vi "SIM Rosenbrock manager.vi"(1 "Simulation data":T1={"continuous integrator"=enum."RK 1 (Euler)", "initial time"=0.0, "final time"=6.0, "step size"=0.0, "proposed step size"=0.001, "max step size"=1e-06, "min step size"=0.0, "discrete time step"=0.0, "max step ratio"=3.0, "Diag Eval Stage"=enum."Major Substep", "Substep Index"=0, "Timestep Index"=10.0, "simulation time"=0.0, "current timestep base"=0.1, "proposed step time"=0.0, "absolute tolerance"=0.0, "relative tolerance"=0.0, "step accepted?"=FALSE, "step complete?"=FALSE, "Halt?"=FALSE, "reset integrator?"=FALSE, "machine epsilon"=1.0, "min float"=0.0, "error"={"status"=FALSE, "code"=0, "source"=""}, "Method Order"=0, "Finished Late [i-1]"=FALSE, "Discrete step?"=FALSE, "NaN and Inf check?"=FALSE, "Final Timestep Index"=0.0, "(maj+disc)or(init)?"=FALSE, "Full Solver Reset"=TRUE, "Execution Mode"=enum."Simulate to Completion", "check vector sizes?"=FALSE, "solver handles zc?"=FALSE, "Simulation Registry"={"Current Idx"=0, "Node Tags"=[], "Node Headers"=[], "Node Data"=[], "Cont State data"={"inputs"=[], "outputs"=[], "reset"=[], "lower limits"=[], "upper limits"=[], "limit types"=[], "reset types"=[], "initial conditions"=[], "reset I.C."=[], "limited?"=[], "State Names"=[]}, "DiscreteInfo"={"tick period (sec)"=0.0, "time (ticks)"=0, "fire?"=[], "registry"={"period (sec)"=[], "skew (sec)"=[], "period (tick)"=[], "skew (tick)"=[]}, "discrete \nblocks?"=FALSE, "steps per tick"=0.0, "steps to tick"=0.0, "discrete \ntick?"=FALSE}, "Disc State data"={"Disc States"=[], "State Names"=[]}, "Registry Error"={"Error Block ID"=0, "code"=0}, "ZC Indices"=[]}, "variable step solver?"=FALSE, "First Substep?"=FALSE, "Continuous States?"=FALSE} {"min float" format="%.1e"; "proposed step size" format="%.1e"; "proposed step time" format="%.1e"; "max step ratio" format="%.1e"; "min step size" format="%.1e"; "machine epsilon" format="%.1e"; "discrete time step" format="%.1e"; "max step size" format="%.1e"; "current timestep base" format="%.1e"; "final time" format="%.1e"; "simulation time" format="%.1e"; "relative tolerance" format="%.1e"; "absolute tolerance" format="%.1e"; "Substep Index" format="%.1e"; "step size" format="%.1e"; "initial time" format="%.1e"}) -> (0 "Simulation data out":T1={"continuous integrator"=enum."RK 1 (Euler)", "initial time"=0.0, "final time"=6.0, "step size"=0.0, "proposed step size"=0.001, "max step size"=1e-06, "min step size"=0.0, "discrete time step"=0.0, "max step ratio"=3.0, "Diag Eval Stage"=enum."Major Substep", "Substep Index"=0, "Timestep Index"=10.0, "simulation time"=0.0, "current timestep base"=0.1, "proposed step time"=0.0, "absolute tolerance"=0.0, "relative tolerance"=0.0, "step accepted?"=FALSE, "step complete?"=FALSE, "Halt?"=FALSE, "reset integrator?"=FALSE, "machine epsilon"=1.0, "min float"=0.0, "error"={"status"=FALSE, "code"=0, "source"=""}, "Method Order"=0, "Finished Late [i-1]"=FALSE, "Discrete step?"=FALSE, "NaN and Inf check?"=FALSE, "Final Timestep Index"=0.0, "(maj+disc)or(init)?"=FALSE, "Full Solver Reset"=TRUE, "Execution Mode"=enum."Simulate to Completion", "check vector sizes?"=FALSE, "solver handles zc?"=FALSE, "Simulation Registry"={"Current Idx"=0, "Node Tags"=[], "Node Headers"=[], "Node Data"=[], "Cont State data"={"inputs"=[], "outputs"=[], "reset"=[], "lower limits"=[], "upper limits"=[], "limit types"=[], "reset types"=[], "initial conditions"=[], "reset I.C."=[], "limited?"=[], "State Names"=[]}, "DiscreteInfo"={"tick period (sec)"=0.0, "time (ticks)"=0, "fire?"=[], "registry"={"period (sec)"=[], "skew (sec)"=[], "period (tick)"=[], "skew (tick)"=[]}, "discrete \nblocks?"=FALSE, "steps per tick"=0.0, "steps to tick"=0.0, "discrete \ntick?"=FALSE}, "Disc State data"={"Disc States"=[], "State Names"=[]}, "Registry Error"={"Error Block ID"=0, "code"=0}, "ZC Indices"=[]}, "variable step solver?"=FALSE, "First Substep?"=FALSE, "Continuous States?"=FALSE} {"min float" format="%.1e"; "proposed step size" format="%.1e"; "proposed step time" format="%.1e"; "max step ratio" format="%.1e"; "min step size" format="%.1e"; "machine epsilon" format="%.1e"; "discrete time step" format="%.1e"; "max step size" format="%.1e"; "current timestep base" format="%.1e"; "final time" format="%.1e"; "simulation time" format="%.1e"; "relative tolerance" format="%.1e"; "absolute tolerance" format="%.1e"; "Substep Index" format="%.1e"; "step size" format="%.1e"; "initial time" format="%.1e"})   [LabVIEW 2020]
uses:
  <vilib>/Simulation/Implementation/Shared/SIM simulation data.ctl
  <vilib>/Simulation/Implementation/Shared/SIM integration method.ctl
  <vilib>/Simulation/Implementation/Shared/SIM diagram eval stage.ctl
  <vilib>/Simulation/Implementation/Shared/SIMSCR Execution Mode.ctl
  <vilib>/Simulation/Implementation/Shared/SIM Registry.llb/SIM Simulation Registry.ctl
  <vilib>/Simulation/Implementation/Shared/SIM Registry.llb/SIM Registry Node Header.ctl
  <vilib>/Simulation/Implementation/Shared/SIM Registry.llb/SIM Registry Node Record.ctl
  <vilib>/Simulation/Implementation/Shared/SIM trigger type.ctl
  <vilib>/Simulation/Implementation/Shared/SIM solver state data.ctl
  <vilib>/Simulation/Implementation/Shared/SIM limit type.ctl
  <vilib>/Simulation/Implementation/Shared/SIM discrete data.ctl
  <vilib>/Simulation/Implementation/Shared/SIM Discrete state data.ctl
  <vilib>/Simulation/Implementation/Shared/SIM Registry.llb/SIM Simulation Registry Error.ctl
  <vilib>/Simulation/ContinuousLinear/Implementation/Shared/Solvers/SIM Rosenbrock.llb/SIM Ros stages.ctl
  <vilib>/Simulation/ContinuousLinear/Implementation/Shared/Solvers/SIM Rosenbrock.llb/SIM Rosenbrock data.ctl
  <vilib>/Simulation/ContinuousLinear/Implementation/Shared/Solvers/SIM Solver Shared.llb/SIM Factored Matrix.ctl
  <vilib>/Simulation/ContinuousLinear/Implementation/Shared/Solvers/SIM BDF.llb/SIM BDF stages.ctl
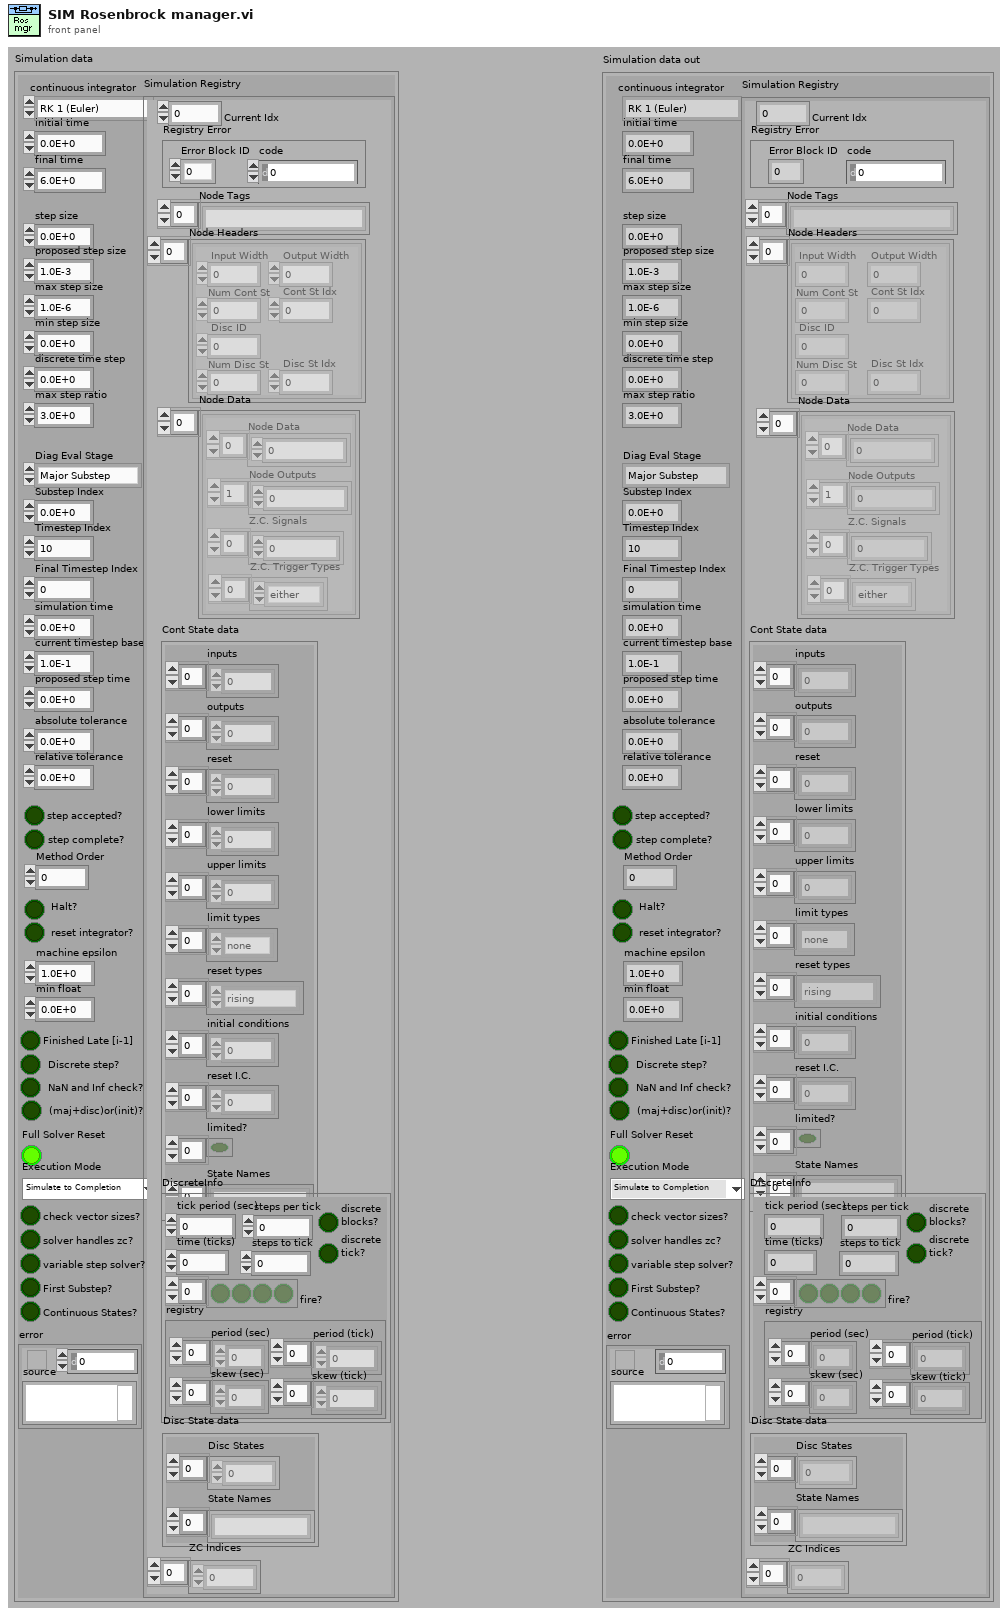
[diagram p1: front panel]
types:
  T1 = typedef "SIM simulation data.ctl" = cluster{"continuous integrator":T2, "initial time":dbl, "final time":dbl, "step size":dbl, "proposed step size":dbl, "max step size":dbl, "min step size":dbl, "discrete time step":dbl, "max step ratio":dbl, "Diag Eval Stage":T3, "Substep Index":i32, "Timestep Index":dbl, "simulation time":dbl, "current timestep base":dbl, "proposed step time":dbl, "absolute tolerance":dbl, "relative tolerance":dbl, "step accepted?":bool, "step complete?":bool, "Halt?":bool, "reset integrator?":bool, "machine epsilon":dbl, "min float":dbl, "error":errorcluster, "Method Order":u32, "Finished Late [i-1]":bool, "Discrete step?":bool, "NaN and Inf check?":bool, "Final Timestep Index":dbl, "(maj+disc)or(init)?":bool, "Full Solver Reset":bool, "Execution Mode":T4, "check vector sizes?":bool, "solver handles zc?":bool, "Simulation Registry":T5, "variable step solver?":bool, "First Substep?":bool, "Continuous States?":bool}
  T2 = typedef "SIM integration method.ctl" = enum16{"RK 1 (Euler)", "Linearizer", "State Query", "Trim Eval", "Adams", "RK 3", "RK 4", "RK 45", "BDF", "RK 2", "RK 23", "Rosenbrock", "Discrete States Only"}
  T3 = typedef "SIM diagram eval stage.ctl" = enum16{"Init", "Minor Substep", "Major Substep", "Final"}
  T4 = typedef "SIMSCR Execution Mode.ctl" = enum16{"Simulate to Completion", "Single Time-Step Simulation (Fixed Step Only)"}
  T5 = typedef "SIM Simulation Registry.ctl" = cluster{"Current Idx":i32, "Node Tags":string[], "Node Headers":T6[], "Node Data":T7[], "Cont State data":T9, "DiscreteInfo":T11, "Disc State data":T12, "Registry Error":T13, "ZC Indices":i32[]}
  T6 = typedef "SIM Registry Node Header.ctl" = cluster{"Input Width":i32, "Disc ID":i32, "Num Cont St":i32, "Cont St Idx":i32, "Num Disc St":i32, "Disc St Idx":i32, "Output Width":i32}
  T7 = typedef "SIM Registry Node Record.ctl" = cluster{"Node Data":dbl[], "Node Outputs":dbl[], "Z.C. Signals":dbl[], "Z.C. Trigger Types":T8[]}
  T8 = typedef "SIM trigger type.ctl" = enum16{"rising", "falling", "either", "none"}
  T9 = typedef "SIM solver state data.ctl" = cluster{"inputs":dbl[], "outputs":dbl[], "reset":dbl[], "lower limits":dbl[], "upper limits":dbl[], "limit types":T10[], "reset types":T8[], "initial conditions":dbl[], "reset I.C.":dbl[], "limited?":bool[], "State Names":string[]}
  T10 = typedef "SIM limit type.ctl" = enum16{"upper", "lower", "both", "none"}
  T11 = typedef "SIM discrete data.ctl" = cluster{"tick period (sec)":dbl, "time (ticks)":i32, "fire?":bool[], "registry":cluster{"period (sec)":dbl[], "skew (sec)":dbl[], "period (tick)":i32[], "skew (tick)":i32[]}, "discrete \nblocks?":bool, "steps per tick":dbl, "steps to tick":dbl, "discrete \ntick?":bool}
  T12 = typedef "SIM Discrete state data.ctl" = cluster{"Disc States":dbl[], "State Names":string[]}
  T13 = typedef "SIM Simulation Registry Error.ctl" = cluster{"Error Block ID":i32, "code":i32}
  T14 = typedef "SIM Ros stages.ctl" = enum16{"Init", "Compute Jacobian", "Compute Ft", "Compute k1", "Compute k2", "Eval Error", "Choose StepSize", "Reset Integrator"}
  T15 = typedef "SIM Rosenbrock data.ctl" = cluster{"y0":dbl[], "F0":dbl[], "F1":dbl[], "k1":dbl[], "k2":dbl[], "Factored W":T16, "Ros Stage":T14, "Ft":dbl[], "Reinit Jac?":bool, "Reinit Ft?":bool, "d":dbl, "e32":dbl}
  T16 = typedef "SIM Factored Matrix.ctl" = cluster{"L":dbl[][], "U":dbl[][], "P":i32[][]}
  T17 = typedef "SIM BDF stages.ctl" = enum16{"Init", "Initial Guess", "Compute Jacobian", "Newton Iteration", "Eval Error", "Choose StepSize", "Reset BDFs"}
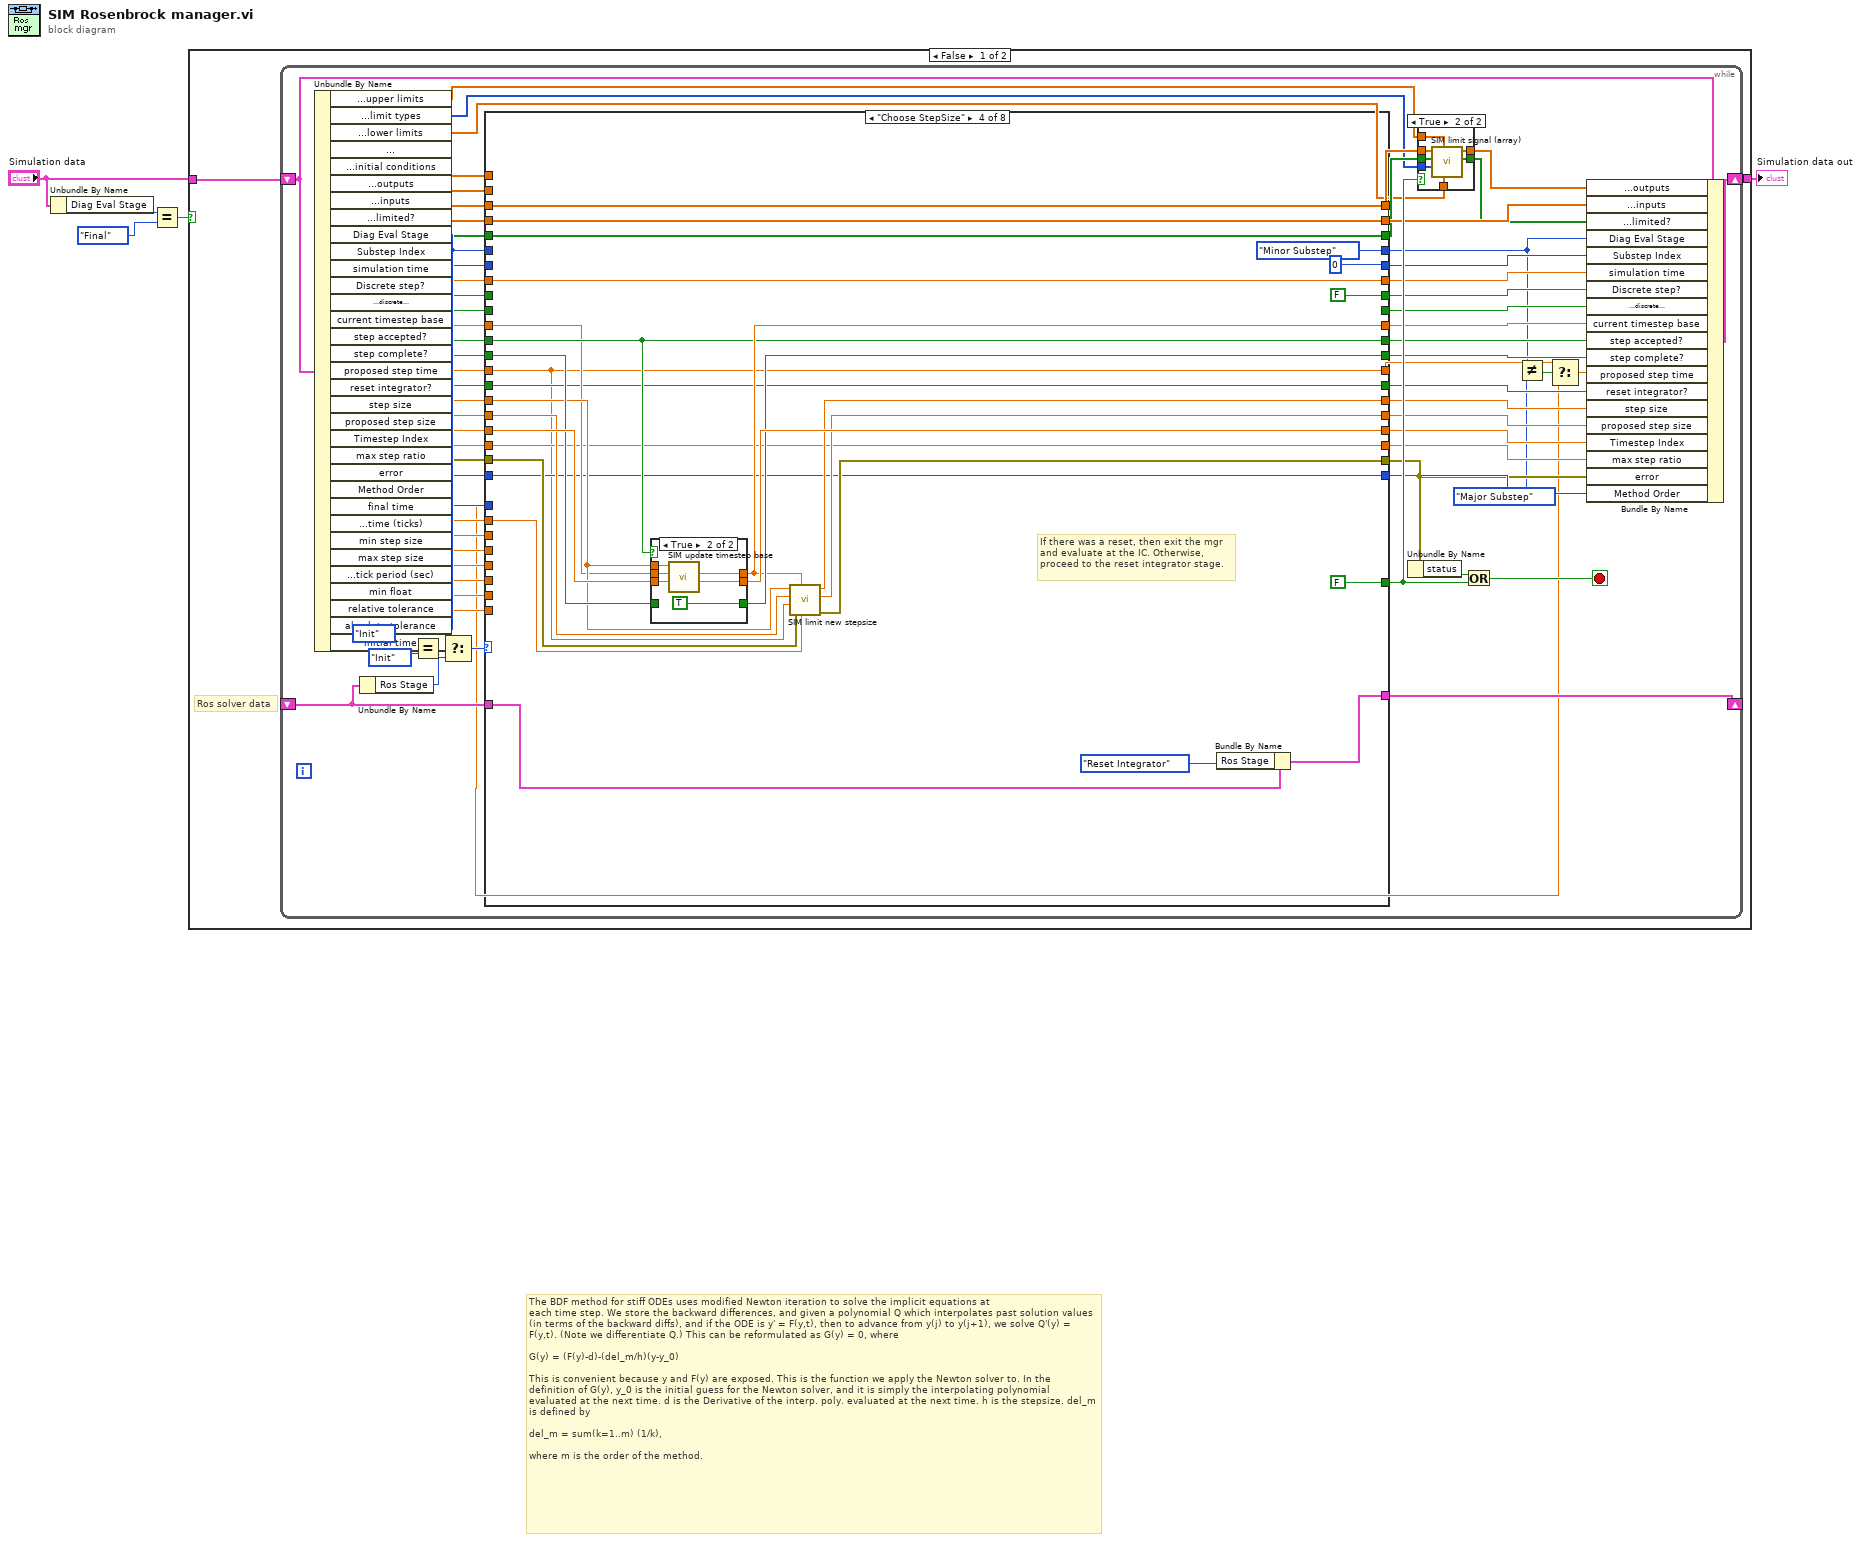
[diagram p0: block diagram]
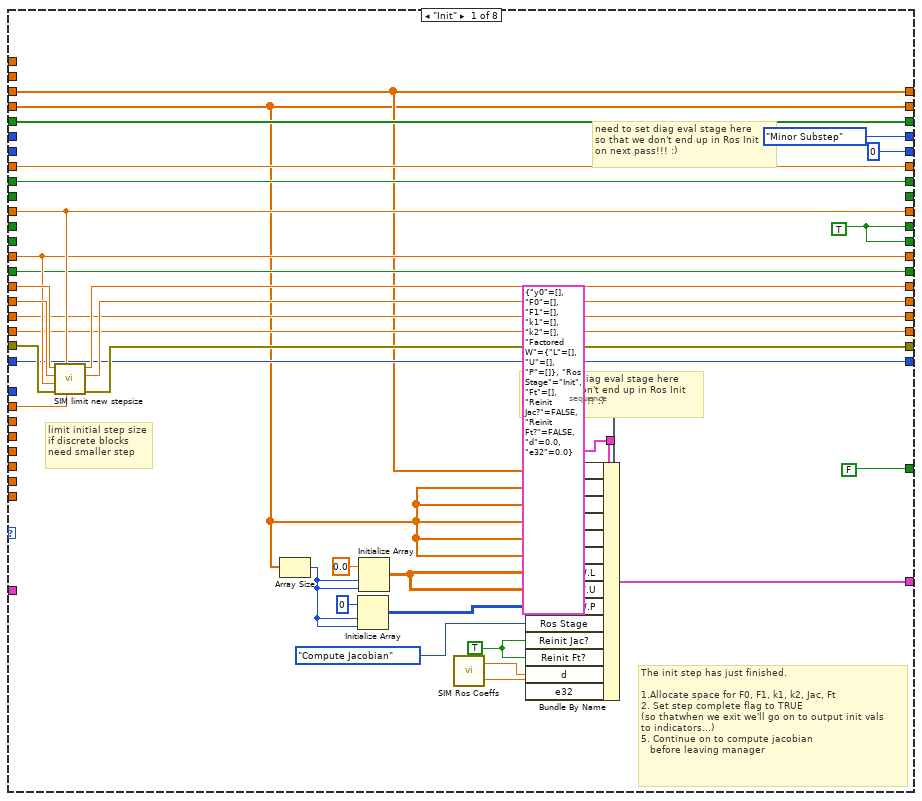
[diagram p3: hidden frame]
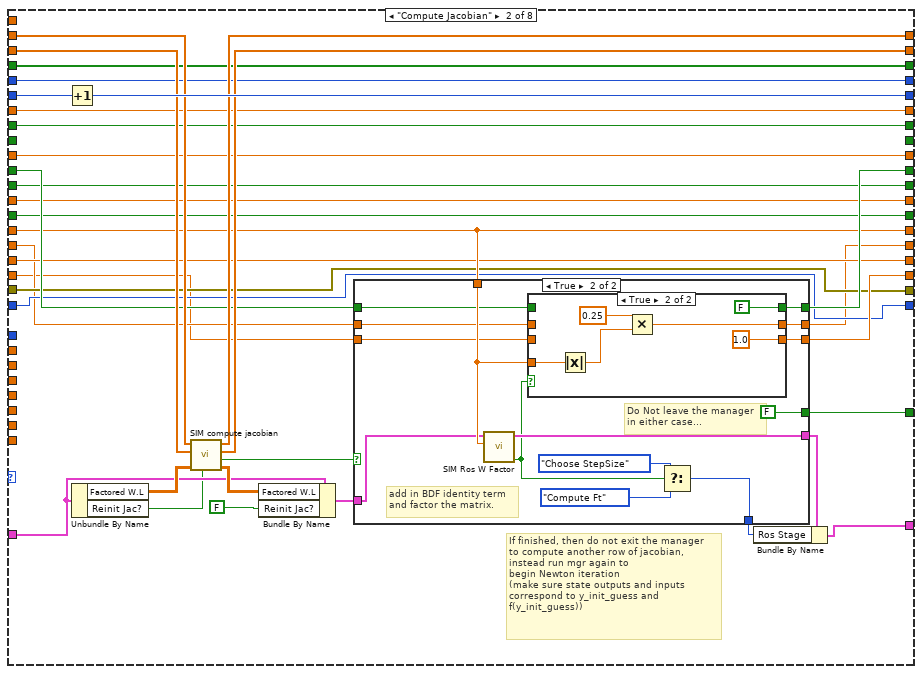
[diagram p4: hidden frame]
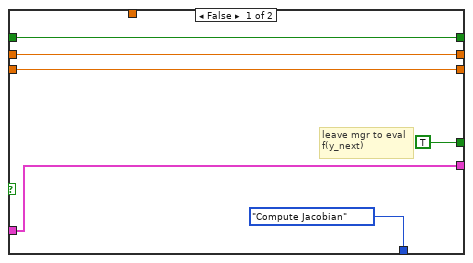
[diagram p5: hidden frame]
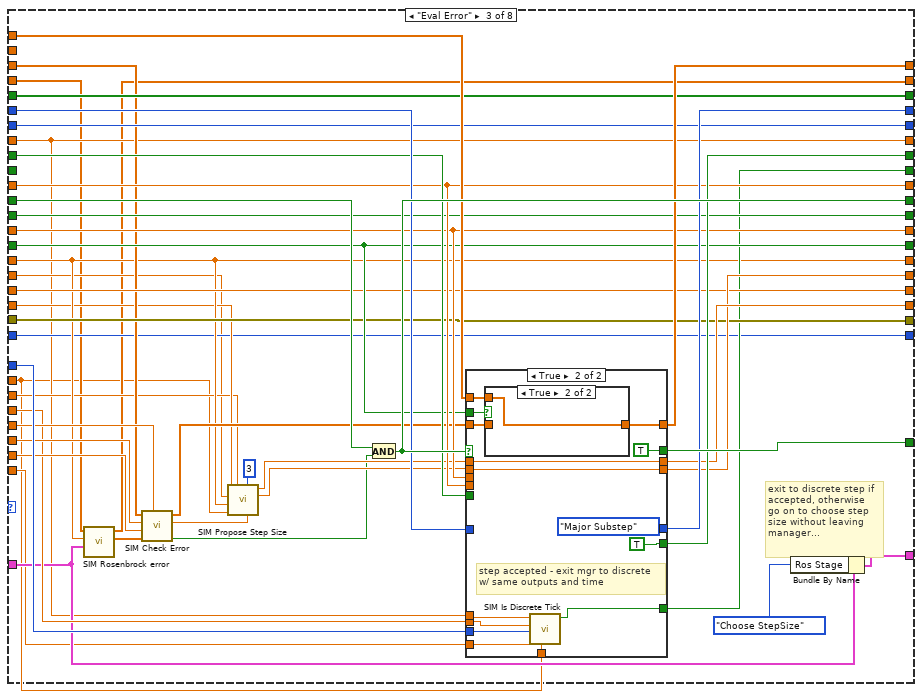
[diagram p7: hidden frame]
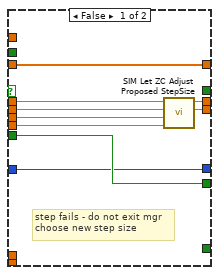
[diagram p8: hidden frame]
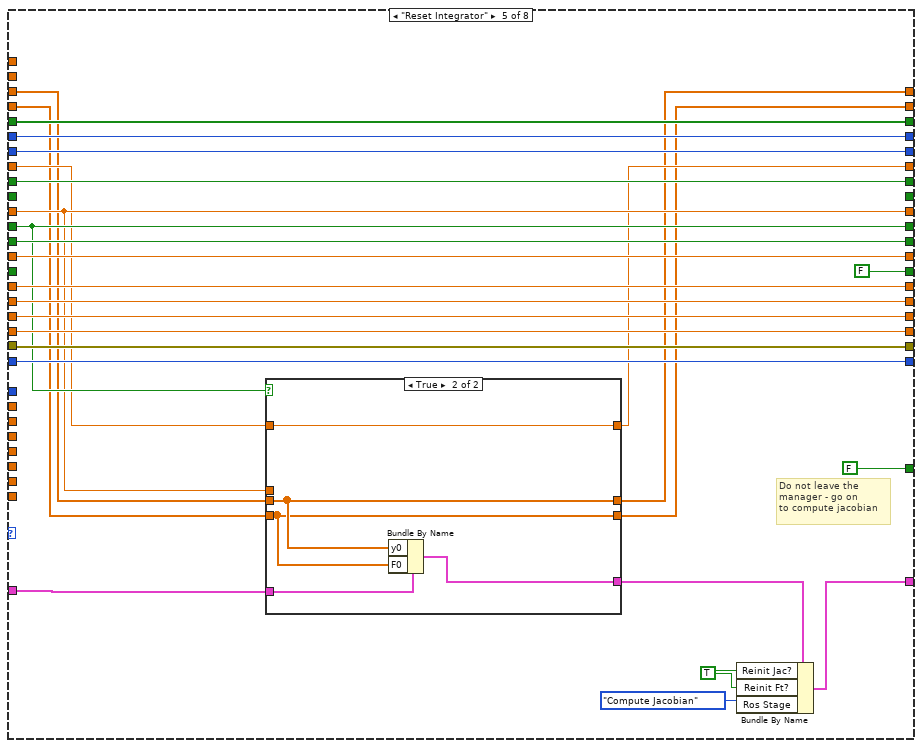
[diagram p11: hidden frame]
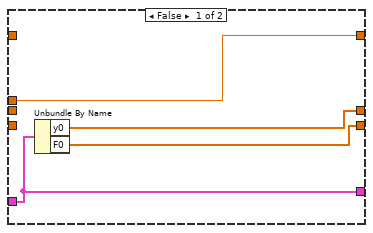
[diagram p12: hidden frame]
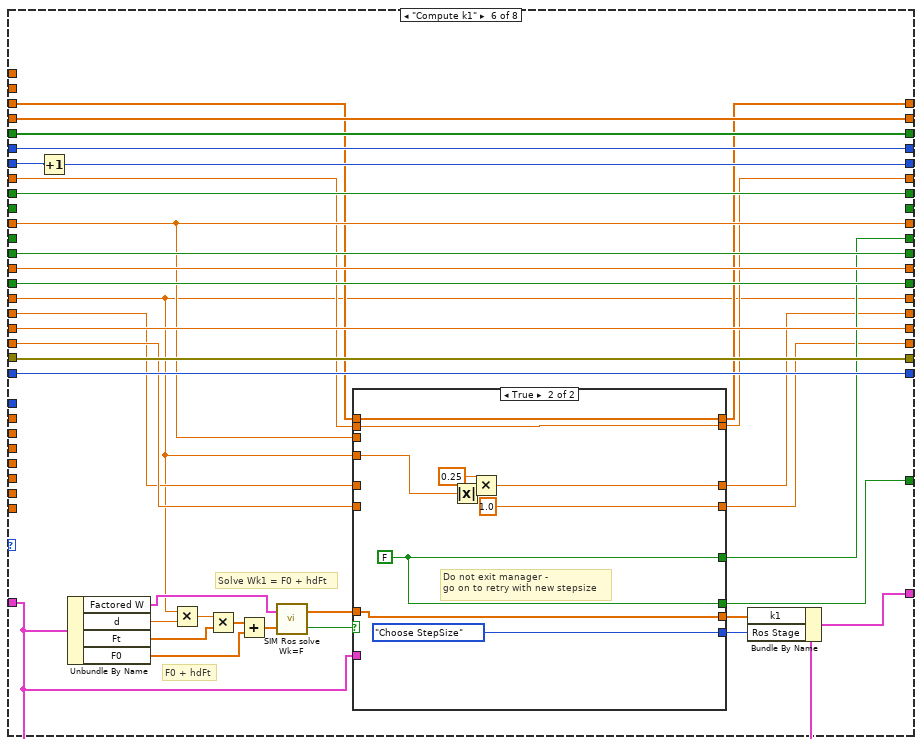
[diagram p13: hidden frame]
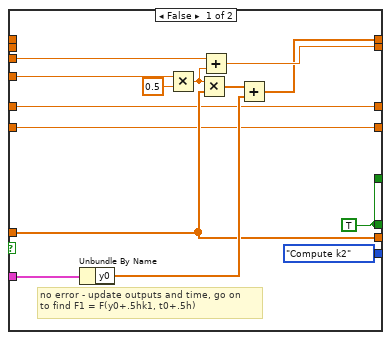
[diagram p14: hidden frame]
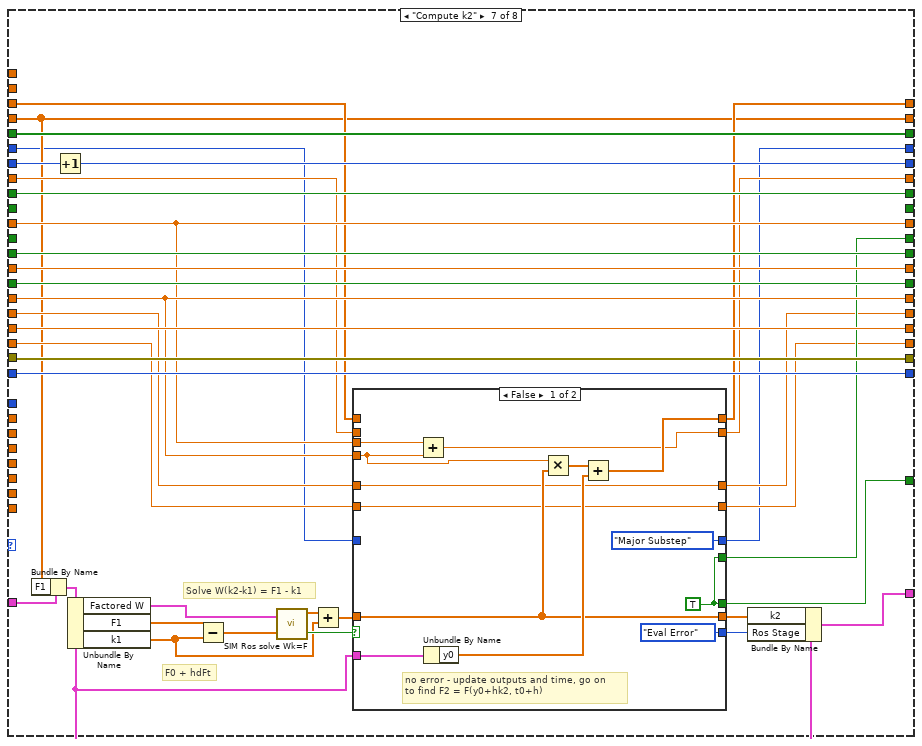
[diagram p15: hidden frame]
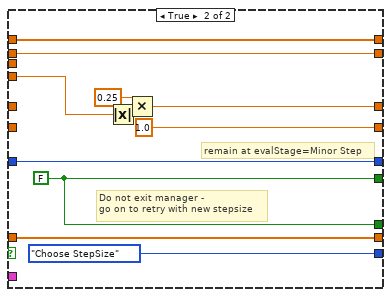
[diagram p16: hidden frame]
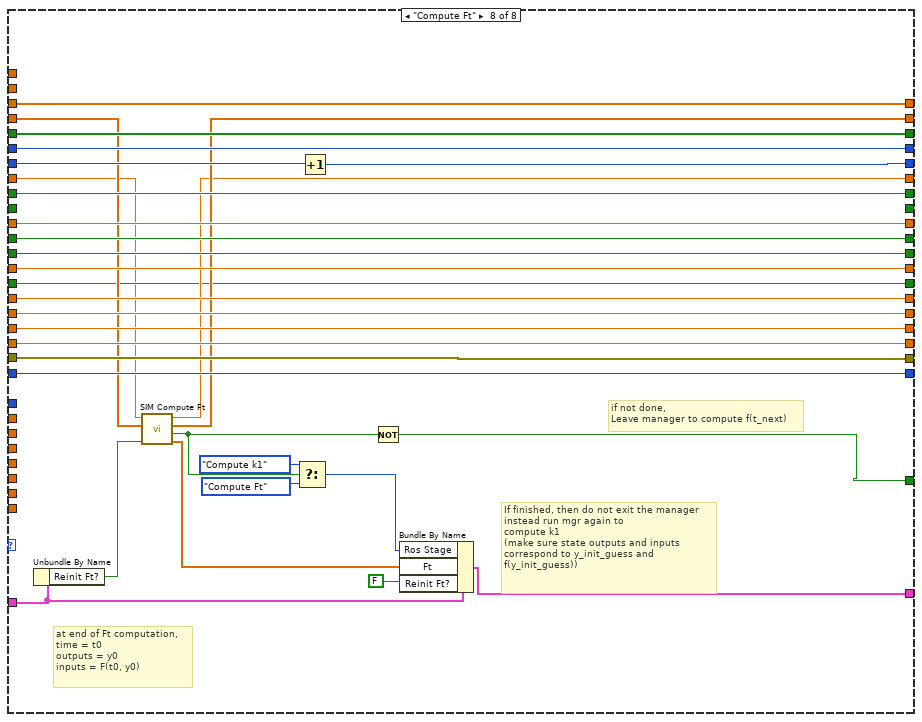
[diagram p17: hidden frame]
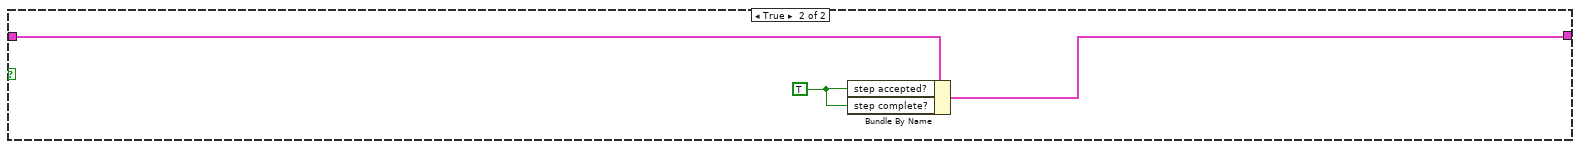
[diagram p18: hidden frame]
diagram:
  # "The BDF method for stiff ODEs uses modified Newton iteration to solve the implicit equations at\neach time step. We store the backward differences, and given a polynomial Q which interpolates past solution values (in terms of the backward diffs), and if the ODE is y' = F(y,t), then to advance from y(j) to y(j+1), we solve Q'(y) = F(y,t). (Note we differentiate Q.) This can be reformulated as G(y) = 0, where \n\nG(y) = (F(y)-d)-(del_m/h)(y-y_0)\n\nThis is convenient because y and F(y) are exposed. This is the function we apply the Newton solver to. In the definition of G(y), y_0 is the initial guess for the Newton solver, and it is simply the interpolating polynomial evaluated at the next time. d is the Derivative of the interp. poly. evaluated at the next time. h is the stepsize. del_m is defined by\n\ndel_m = sum(k=1..m) (1/k),\n\nwhere m is the order of the method."
  n1 = Unbundle By Name("Simulation data") -> ("Diag Eval Stage"=w3:T3)
  n2 = Equal?(x=w3, y=SIM_diagram_eval_stage."Final") -> (x = y?=w1:bool)
  n3 = case shown="False" w1 {
    tunnel: [w7 w484] -> w5
    tunnel: "Simulation data" -> [w6 w483]
    frame False {
      # "Ros solver data"
      n4 = while {
        shift-right: [w38] -> w7
        shift-left: w6 -> [w18]
        shift-right: [w16] -> _
        shift-left: _ -> [w73]
        stop <- w74 stop-if-true
        n5 = Unbundle By Name(w18) -> ("Simulation Registry.Cont State data.upper limits"=w21:dbl[], "Simulation Registry.Cont State data.limit types"=w19:T10[], "Simulation Registry.Cont State data.lower limits"=w20:dbl[], "Simulation Registry.Cont State data.reset I.C."=w30:dbl[], "Simulation Registry.Cont State data.initial conditions"=w33:dbl[], "Simulation Registry.Cont State data.outputs"=w42:dbl[], "Simulation Registry.Cont State data.inputs"=w41:dbl[], "Simulation Registry.Cont State data.limited?"=w35:bool[], "Diag Eval Stage"=w68:T3, "Substep Index"=w67:i32, "simulation time"=w65:dbl, "Discrete step?"=w63:bool, "Simulation Registry.DiscreteInfo.discrete \ntick?"=w61:bool, "current timestep base"=w59:dbl, "step accepted?"=w57:bool, "step complete?"=w55:bool, "proposed step time"=w53:dbl, "reset integrator?"=w52:bool, "step size"=w50:dbl, "proposed step size"=w48:dbl, "Timestep Index"=w46:dbl, "max step ratio"=w44:dbl, "error"=w28:errorcluster, "Method Order"=w27:u32, "final time"=w8:dbl, "Simulation Registry.DiscreteInfo.time (ticks)"=w17:i32, "min step size"=w34:dbl, "max step size"=w31:dbl, "Simulation Registry.DiscreteInfo.tick period (sec)"=w39:dbl, "min float"=w32:dbl, "relative tolerance"=w37:dbl, "absolute tolerance"=w36:dbl, "initial time"=w14:dbl)
        n6 = Unbundle By Name(w73) -> ("Ros Stage"=w72:T14)
        n7 = Equal?(x=w68, y=SIM_diagram_eval_stage."Init") -> (x = y?=w70:bool)
        n8 = Select(t=SIM_Ros_stages."Init" ("Ros Stage"), s=w70, f=w72) -> (s? t:f=w75:T14)
        n9 = case shown="\"Choose StepSize\"" w75 {
          tunnel: [FALSE w148 w229 FALSE ("finished?") FALSE ("finished?") w343 w412 w454] -> w69
          tunnel: w73 -> [_ w152 w193 w263 w306 w332 w401 w465]
          tunnel: [SIM_diagram_eval_stage."Minor Substep" ("Diag Eval Stage") w141 w225 SIM_diagram_eval_stage."Minor Substep" ("Diag Eval Stage") w318 w364 w391 w480] -> w9
          tunnel: w68 -> [_ w141 w221 _ w318 w364 w392 w480]
          tunnel: [0 ("Substep Index") w146 w217 0 ("Substep Index") w317 w345 w415 w467] -> w66
          tunnel: w67 -> [_ w147 w217 _ w317 w346 w416 w468]
          tunnel: w65 -> [w107 w137 w189 w270 w303 w340 w409 w452]
          tunnel: [w107 w137 w189 w270 w304 w339 w408 w456] -> w64
          tunnel: [w106 w136 w224 FALSE ("Discrete step?") w316 w363 w426 w479] -> w62
          tunnel: w63 -> [w106 w136 w220 _ w316 w363 w426 w479]
          tunnel: w61 -> [_ _ _ _ _ _ _ _]
          tunnel: [_ _ w209 _ _ _ _ _] -> w60
          tunnel: [w105 w135 w216 w273 w305 w341 w410 w478] -> w58
          tunnel: w59 -> [w105 w135 w216 w268 w305 w341 w410 w478]
          tunnel: [w110 w139 w227 w269 w307 w342 w411 w477] -> w56
          tunnel: w57 -> [_ w138 w228 w269 w307 _ _ w477]
          tunnel: [w110 w134 w215 w281 w315 w362 w425 w476] -> w54
          tunnel: w55 -> [_ w134 w215 w282 w315 w362 w425 w476]
          tunnel: [w104 w127 w214 w259 w314 w361 w424 w475] -> w10
          tunnel: w53 -> [w104 w127 w214 w259 w314 w361 w424 w475]
          tunnel: [w103 w133 w213 w267 FALSE ("reset integrator?") w344 w414 w453] -> w51
          tunnel: w52 -> [w103 w133 w213 w267 _ w344 w414 w453]
          tunnel: [w111 w132 w199 w275 w313 w330 w413 w474] -> w49
          tunnel: w50 -> [w117 w132 w199 w274 w313 w330 w413 w474]
          tunnel: [w113 w126 w222 w277 w312 w334 w403 w473] -> w47
          tunnel: w48 -> [w116 w125 w190 w280 w312 w333 w402 w473]
          tunnel: [w102 w131 w212 w283 w311 w360 w423 w472] -> w45
          tunnel: w46 -> [w102 w131 w212 w284 w311 w360 w423 w472]
          tunnel: [w101 w140 w223 w265 w310 w336 w405 w471] -> w43
          tunnel: w44 -> [w101 w124 w198 w265 w310 w335 w404 w471]
          tunnel: w42 -> [w89 w145 w206 w258 w302 w337 w406 w482]
          tunnel: w41 -> [w88 w144 w188 w272 w295 w366 w400 w458]
          tunnel: [w89 w143 w219 w258 w301 w338 w407 w482] -> w25
          tunnel: [w88 w142 w187 w272 w300 w366 w400 w457] -> w40
          tunnel: w39 -> [_ _ w200 _ _ _ _ _]
          tunnel: w37 -> [_ _ w204 _ _ _ _ _]
          tunnel: w36 -> [_ _ w203 _ _ _ _ _]
          tunnel: w35 -> [w108 w128 w218 w271 w319 w365 w427 w481]
          tunnel: w28 -> [w115 w130 w211 w279 w309 w359 w422 w470]
          tunnel: w34 -> [w114 _ w185 w278 _ _ _ _]
          tunnel: [w112 w130 w211 w276 w309 w359 w422 w470] -> w26
          tunnel: w33 -> [_ _ _ _ _ _ _ _]
          tunnel: [w108 w128 w218 w271 w319 w365 w427 w481] -> w22
          tunnel: w32 -> [_ _ w208 _ _ _ _ _]
          tunnel: w31 -> [_ _ w197 _ _ _ _ _]
          tunnel: w30 -> [_ _ w226 _ _ _ _ _]
          tunnel: [w100 w129 w191 w266 w308 w358 w421 w469] -> w29
          tunnel: w27 -> [w100 w129 w191 w266 w308 w358 w421 w469]
          tunnel: w17 -> [_ _ w210 _ _ _ _ _]
          tunnel: [w87 w120 w192 w262 w297 w331 w397 w463] -> w16
          tunnel: w14 -> [_ _ w186 _ _ _ _ _]
          frame "Init" {
            w90 = TRUE ("Reinit Jac?")
            w110 = TRUE ("step complete?")
            # "limit initial step size\nif discrete blocks\nneed smaller step"
            # "need to set diag eval stage here\nso that we don't end up in Ros Init\non next pass!!! :)"
            # "need to set diag eval stage here\nso that we don't end up in Ros Init\non next pass!!! :)"
            # "The init step has just finished.\n\n1.Allocate space for F0, F1, k1, k2, Jac, Ft\n2. Set step complete flag to TRUE\n(so thatwhen we exit we'll go on to output init vals\nto indicators...)\n5. Continue on to compute jacobian\n   before leaving manager"
            n10 = call <vilib>:"SIM limit new stepsize.vi"("min step size"=w114, "current timestep base"=w105, "error"=w115, "proposed step time"=w104, "proposed step size"=w116, "step size"=w117) -> ("error out"=w112:errorcluster, "proposed step size"=w113:dbl, "step size"=w111:dbl)  [unwired: 3 out]
            n11 = Array Size(array=w88) -> (size(s)=w96:i32)
            n12 = Initialize Array(0 ("element"), w96, w96) -> (w95:i32[][])
            n13 = Initialize Array(0.0 ("element"), w96, w96) -> (w94:dbl[][])
            n14 = call <vilib>:"SIM Ros Coeffs.vi"() -> ("e32"=w91:dbl, "d"=w92:dbl)
            n15 = stacked-sequence {
              tunnel: [T15 {"y0"=[], "F0"=[], "F1"=[], "k1"=[], "k2"=[], "Factored W"={"L"=[], "U"=[], "P"=[]}, "Ros Stage"=enum."Init", "Ft"=[], "Reinit Jac?"=FALSE, "Reinit Ft?"=FALSE, "d"=0.0, "e32"=0.0} ("BDF data")] -> w99
              frame #0 {
              }
            }
            n16 = Bundle By Name(cluster=w99, "y0"=w89, "F0"=w88, "F1"=w88, "k1"=w88, "k2"=w88, "Ft"=w88, "Factored W.L"=w94, "Factored W.U"=w94, "Factored W.P"=w95, "Ros Stage"=SIM_Ros_stages."Compute Jacobian", "Reinit Jac?"=w90, "Reinit Ft?"=w90, "d"=w92, "e32"=w91) -> (w87:T15)
          }
          frame "Compute Jacobian" {
            # "If finished, then do not exit the manager\nto compute another row of jacobian,\ninstead run mgr again to \nbegin Newton iteration\n(make sure state outputs and inputs\ncorrespond to y_init_guess and\nf(y_init_guess))"
            n17 = Increment(x=w147) -> (x+1=w146:i32)
            n18 = Unbundle By Name(w152) -> ("Factored W.L"=w154:dbl[][], "Reinit Jac?"=w123:bool)
            n19 = call <vilib>:"SIM compute jacobian.vi"("reset?"=w123, "Current jacobian"=w154, "F(y)"=w144, "y current"=w145) -> ("Current jacobian out"=w153:dbl[][], "finished?"=w151:bool, "F(y_0)"=w142:dbl[], "y next"=w143:dbl[])  [unwired: 2 in, 2 out]
            n20 = Bundle By Name(cluster=w152, "Factored W.L"=w153, "Reinit Jac?"=FALSE ("need jac module re-init")) -> (w150:T15)
            n21 = case shown="True" w151 {
              tunnel: w150 -> [w156 w164]
              tunnel: [w156 w173] -> w149
              tunnel: [TRUE FALSE] -> w148
              tunnel: w132 -> [_ w171]
              tunnel: [w158 w170] -> w126
              tunnel: [w159 w169] -> w140
              tunnel: [w157 w168] -> w139
              tunnel: w124 -> [w159 w166]
              tunnel: w125 -> [w158 w165]
              tunnel: w138 -> [w157 w167]
              tunnel: [SIM_Ros_stages."Compute Jacobian" ("Enum") w163] -> w121
              frame False {
                (unwired) SIM_BDF_stages."Compute Jacobian" ("Enum")
                # "leave mgr to eval\nf(y_next)"
              }
              frame True {
                # "Do Not leave the manager\nin either case..."
                # "add in BDF identity term\nand factor the matrix."
                n22 = call <vilib>:"SIM Ros W Factor.vi"("step size"=w171, "Ros data"=w164) -> ("error"=w172:bool, "Ros data out"=w173:T15)  [unwired: 1 in, 7 out]
                n23 = case shown="True" w172 {
                  tunnel: w171 -> [_ w181]
                  tunnel: [w175 w180] -> w170
                  tunnel: [w176 1.0 ("max step ratio")] -> w169
                  tunnel: [w177 FALSE ("step accepted?")] -> w168
                  tunnel: w167 -> [w177 _]
                  tunnel: w166 -> [w176 _]
                  tunnel: w165 -> [w175 _]
                  frame False {
                  }
                  frame True {
                    n24 = Absolute Value(x=w181) -> (abs(x)=w182:dbl)
                    n25 = Multiply(x=0.25, y=w182) -> (x*y=w180:dbl)
                  }
                }
                n26 = Select(t=SIM_Ros_stages."Choose StepSize", s=w172, f=SIM_Ros_stages."Compute Ft" ("Enum")) -> (s? t:f=w163:T14)
              }
            }
            n27 = Bundle By Name(cluster=w149, "Ros Stage"=w121) -> (w120:T15)
          }
          frame "Eval Error" {
            # "exit to discrete step if\naccepted, otherwise\ngo on to choose step \nsize without leaving\nmanager..."
            n28 = call <vilib>:"SIM Rosenbrock error.vi"("Ros data"=w193, "step size"=w199, "F2"=w188) -> ("error"=w207:dbl[], "F2 out"=w187:dbl[])  [unwired: 5 out]
            n29 = call <vilib>:"SIM Check Error.vi"("min float"=w208, "estimated error"=w207, "absolute tolerance"=w203, "relative tolerance"=w204, "Solution"=w206) -> ("within acceptable err?"=w194:bool, "acceptable err/estimated err"=w201:dbl, "Solution Out"=w205:dbl[])  [unwired: 4 out]
            n30 = call <vilib>:"SIM Propose Step Size.vi"("acceptable err/estimated err"=w201, "error order"=3, "max step size"=w197, "min step size"=w185, "step size"=w199, "proposed step size"=w190, "max step ratio"=w198) -> ("proposed step size out"=w196:dbl, "proposed max step ratio"=w195:dbl)  [unwired: 3 out]
            n31 = And(x=w228, y=w194) -> (x .and. y?=w227:bool)
            n32 = case shown="True" w227 {
              tunnel: w213 -> [_ w253]
              tunnel: [_ TRUE] -> w229
              tunnel: w226 -> [_ w251]
              tunnel: [w238 w250] -> w219
              tunnel: w205 -> [w238 w249]
              tunnel: [w230 SIM_diagram_eval_stage."Major Substep" ("Diag Eval Stage")] -> w225
              tunnel: [w231 TRUE ("Discrete step?")] -> w224
              tunnel: [w237 w245] -> w223
              tunnel: [w236 w246] -> w222
              tunnel: w195 -> [w235 w245]
              tunnel: w196 -> [w234 w246]
              tunnel: w214 -> [w233 _]
              tunnel: w216 -> [w232 _]
              tunnel: w221 -> [w230 _]
              tunnel: w220 -> [w231 _]
              tunnel: w200 -> [_ w243]
              tunnel: w210 -> [_ w242]
              tunnel: [_ w239] -> w209
              tunnel: w189 -> [_ w244]
              tunnel: w186 -> [_ w241]
              tunnel: w185 -> [_ w240]
              frame False {
                # "step fails - do not exit mgr\nchoose new step size"
                n33 = call <vilib>:"SIM Let ZC Adjust Proposed StepSize.vi"("current timestep base"=w232, "proposed step time"=w233, "proposed step size"=w234, "max step ratio"=w235) -> ("proposed step size out"=w236:dbl, "max step ratio out"=w237:dbl)  [unwired: 2 out]
              }
              frame True {
                (unwired) TRUE
                # "step accepted - exit mgr to discrete\nw/ same outputs and time"
                n34 = case shown="True" w253 {
                  tunnel: w251 -> [_ w255]
                  tunnel: [w254 w255] -> w250
                  tunnel: w249 -> [w254 _]
                  frame False {
                  }
                  frame True {
                  }
                }
                n35 = call <vilib>:"SIM Is Discrete Tick.vi"("min step size"=w240, "initial time"=w241, "time (ticks)"=w242, "tick period (sec)"=w243, "simulation time"=w244) -> ("Discrete Tick?"=w239:bool)  [unwired: 6 out]
              }
            }
            n36 = Bundle By Name(cluster=w193, "Ros Stage"=SIM_Ros_stages."Choose StepSize") -> (w192:T15)
          }
          frame "Choose StepSize" {
            # "If there was a reset, then exit the mgr\nand evaluate at the IC. Otherwise, \nproceed to the reset integrator stage."
            n37 = case shown="True" w269 {
              tunnel: w274 -> [_ w293]
              tunnel: w268 -> [w287 w292]
              tunnel: w284 -> [w286 w291]
              tunnel: [w287 w290] -> w273
              tunnel: [w286 w289] -> w283
              tunnel: [w285 TRUE ("step complete?")] -> w281
              tunnel: w282 -> [w285 _]
              frame False {
              }
              frame True {
                n38 = call <vilib>:"SIM update timestep base.vi"("Timestep Index"=w291, "current timestep base"=w292, "step size"=w293) -> ("Timestep Index out"=w289:dbl, "current timestep base out"=w290:dbl)  [unwired: 3 out]
              }
            }
            n39 = call <vilib>:"SIM limit new stepsize.vi"("min step size"=w278, "current timestep base"=w273, "error"=w279, "proposed step time"=w259, "proposed step size"=w280, "step size"=w274) -> ("error out"=w276:errorcluster, "proposed step size"=w277:dbl, "step size"=w275:dbl)  [unwired: 3 out]
            n40 = Bundle By Name(cluster=w263, "Ros Stage"=SIM_Ros_stages."Reset Integrator") -> (w262:T15)
          }
          frame "Reset Integrator" {
            w298 = TRUE ("Reinit Ft?")
            # "Do not leave the\nmanager - go on\nto compute jacobian"
            n41 = case shown="True" w307 {
              tunnel: [w324 w329] -> w296
              tunnel: w306 -> [w324 w328]
              tunnel: w302 -> [_ w326]
              tunnel: w295 -> [_ w325]
              tunnel: w305 -> [w323 _]
              tunnel: [w323 w327] -> w304
              tunnel: w303 -> [_ w327]
              tunnel: [w322 w326] -> w301
              tunnel: [w321 w325] -> w300
              frame False {
                n42 = Unbundle By Name(w324) -> ("y0"=w322:dbl[], "F0"=w321:dbl[])
              }
              frame True {
                n43 = Bundle By Name(cluster=w328, "y0"=w326, "F0"=w325) -> (w329:T15)
              }
            }
            n44 = Bundle By Name(cluster=w296, "Reinit Jac?"=w298, "Reinit Ft?"=w298, "Ros Stage"=SIM_Ros_stages."Compute Jacobian" ("BDF stage")) -> (w297:T15)
          }
          frame "Compute k1" {
            # "Solve Wk1 = F0 + hdFt"
            # "F0 + hdFt"
            n45 = Increment(x=w346) -> (x+1=w345:i32)
            n46 = Unbundle By Name(w332) -> ("Factored W"=w351:T16, "d"=w357:dbl, "Ft"=w355:dbl[], "F0"=w353:dbl[])
            n47 = Multiply(x=w330, y=w357) -> (x*y=w356:dbl)
            n48 = Multiply(x=w356, y=w355) -> (x*y=w354:dbl[])
            n49 = Add(x=w354, y=w353) -> (x+y=w352:dbl[])
            n50 = call <vilib>:"SIM Ros solve Wk=F.vi"("F"=w352, "Factored W"=w351) -> ("Error?"=w350:bool, "k"=w349:dbl[])
            n51 = case shown="True" w350 {
              tunnel: [w374 w385] -> w343
              tunnel: w349 -> [w369 w390]
              tunnel: [w369 w390] -> w348
              tunnel: [SIM_Ros_stages."Compute k2" ("Ros Stage") SIM_Ros_stages."Choose StepSize" ("Ros Stage")] -> w347
              tunnel: w332 -> [w376 _]
              tunnel: w330 -> [w372 w386]
              tunnel: [w374 w385] -> w342
              tunnel: w341 -> [w373 _]
              tunnel: [w371 w384] -> w339
              tunnel: w340 -> [_ w384]
              tunnel: [w370 w383] -> w338
              tunnel: w337 -> [_ w383]
              tunnel: [w368 1.0 ("max step ratio")] -> w336
              tunnel: w335 -> [w368 _]
              tunnel: [w367 w381] -> w334
              tunnel: w333 -> [w367 _]
              frame False {
                w374 = TRUE
                # "no error - update outputs and time, go on\nto find F1 = F(y0+.5hk1, t0+.5h)"
                n52 = Unbundle By Name(w376) -> ("y0"=w375:dbl[])
                n53 = Multiply(x=w372, y=0.5) -> (x*y=w379:dbl)
                n54 = Multiply(x=w379, y=w369) -> (x*y=w377:dbl[])
                n55 = Add(x=w373, y=w379) -> (x+y=w371:dbl)
                n56 = Add(x=w377, y=w375) -> (x+y=w370:dbl[])
              }
              frame True {
                w385 = FALSE
                # "Do not exit manager - \ngo on to retry with new stepsize"
                n57 = Absolute Value(x=w386) -> (abs(x)=w387:dbl)
                n58 = Multiply(x=0.25, y=w387) -> (x*y=w381:dbl)
              }
            }
            n59 = Bundle By Name(cluster=w332, "k1"=w348, "Ros Stage"=w347) -> (w331:T15)
          }
          frame "Compute k2" {
            # "Solve W(k2-k1) = F1 - k1"
            # "F0 + hdFt"
            n60 = Bundle By Name(cluster=w401, "F1"=w400) -> (w393:T15)
            n61 = Increment(x=w416) -> (x+1=w415:i32)
            n62 = Unbundle By Name(w393) -> ("Factored W"=w420:T16, "F1"=w399:dbl[], "k1"=w395:dbl[])
            n63 = Subtract(x=w399, y=w395) -> (x-y=w398:dbl[])
            n64 = call <vilib>:"SIM Ros solve Wk=F.vi"("F"=w398, "Factored W"=w420) -> ("Error?"=w419:bool, "k"=w396:dbl[])
            n65 = Add(x=w396, y=w395) -> (x+y=w394:dbl[])
            n66 = case shown="False" w419 {
              tunnel: [w436 w446] -> w412
              tunnel: w394 -> [w433 w451]
              tunnel: [w433 w451] -> w418
              tunnel: [SIM_Ros_stages."Eval Error" ("Ros Stage") SIM_Ros_stages."Choose StepSize" ("Ros Stage")] -> w417
              tunnel: w393 -> [w438 _]
              tunnel: w413 -> [w429 w447]
              tunnel: [w436 w446] -> w411
              tunnel: w410 -> [w435 _]
              tunnel: [w430 w445] -> w408
              tunnel: w409 -> [_ w445]
              tunnel: [w434 w444] -> w407
              tunnel: w406 -> [_ w444]
              tunnel: [w432 1.0 ("max step ratio")] -> w405
              tunnel: w404 -> [w432 _]
              tunnel: [w431 w442] -> w403
              tunnel: w402 -> [w431 _]
              tunnel: w392 -> [_ w441]
              tunnel: [SIM_diagram_eval_stage."Major Substep" ("Diag Eval Stage") w441] -> w391
              frame False {
                w436 = TRUE
                # "no error - update outputs and time, go on\nto find F2 = F(y0+hk2, t0+h)"
                n67 = Add(x=w435, y=w429) -> (x+y=w430:dbl)
                n68 = Unbundle By Name(w438) -> ("y0"=w437:dbl[])
                n69 = Multiply(x=w429, y=w433) -> (x*y=w439:dbl[])
                n70 = Add(x=w439, y=w437) -> (x+y=w434:dbl[])
              }
              frame True {
                w446 = FALSE
                # "remain at evalStage=Minor Step"
                # "Do not exit manager - \ngo on to retry with new stepsize"
                n71 = Absolute Value(x=w447) -> (abs(x)=w448:dbl)
                n72 = Multiply(x=0.25, y=w448) -> (x*y=w442:dbl)
              }
            }
            n73 = Bundle By Name(cluster=w393, "k2"=w418, "Ros Stage"=w417) -> (w397:T15)
          }
          frame "Compute Ft" {
            # "if not done, \nLeave manager to compute f(t_next)"
            # "at end of Ft computation,\ntime = t0\noutputs = y0\ninputs = F(t0, y0)"
            # "If finished, then do not exit the manager\ninstead run mgr again to \ncompute k1\n(make sure state outputs and inputs\ncorrespond to y_init_guess and\nf(y_init_guess))"
            n74 = Unbundle By Name(w465) -> ("Reinit Ft?"=w466:bool)
            n75 = call <vilib>:"SIM Compute Ft.vi"("reset?"=w466, "F_current"=w458, "t_current"=w452) -> ("Ft"=w462:dbl[], "done?"=w455:bool, "F0"=w457:dbl[], "t_next"=w456:dbl)  [unwired: 1 out]
            n76 = Select(t=SIM_Ros_stages."Compute k1", s=w455, f=SIM_Ros_stages."Compute Ft" ("Ros Stage")) -> (s? t:f=w459:T14)
            n77 = Increment(x=w468) -> (x+1=w467:i32)
            n78 = Not(x=w455) -> (.not. x?=w454:bool)
            n79 = Bundle By Name(cluster=w465, "Ros Stage"=w459, "Ft"=w462, "Reinit Ft?"=FALSE) -> (w463:T15)
          }
        }
        n80 = Unbundle By Name(w26) -> ("status"=w71:bool)
        n81 = case shown="True" w69 {
          tunnel: w25 -> [w78 w85]
          tunnel: [w78 w84] -> w24
          tunnel: [w77 w83] -> w23
          tunnel: w22 -> [w77 w82]
          tunnel: w21 -> [_ w81]
          tunnel: w20 -> [_ w80]
          tunnel: w19 -> [_ w79]
          frame False {
          }
          frame True {
            n82 = call <vilib>:"SIM limit signal (array).vi"("lower limits"=w80, "upper limits"=w81, "limit types"=w79, "limited? in"=w82, "inputs"=w85) -> ("limited? out"=w83:bool[], "outputs"=w84:dbl[])  [unwired: 1 in, 4 out]
          }
        }
        n83 = Or(x=w71, y=w69) -> (x .or. y?=w74:bool)
        n84 = Not Equal?(x=w9, y=SIM_diagram_eval_stage."Major Substep") -> (x != y?=w11:bool)
        n85 = Select(t=w10, s=w11, f=w8) -> (s? t:f=w12:dbl)
        n86 = Bundle By Name(cluster=w18, "Simulation Registry.Cont State data.outputs"=w24, "Simulation Registry.Cont State data.inputs"=w40, "Simulation Registry.Cont State data.limited?"=w23, "Diag Eval Stage"=w9, "Substep Index"=w66, "simulation time"=w64, "Discrete step?"=w62, "Simulation Registry.DiscreteInfo.discrete \ntick?"=w60, "current timestep base"=w58, "step accepted?"=w56, "step complete?"=w54, "proposed step time"=w12, "reset integrator?"=w51, "step size"=w49, "proposed step size"=w47, "Timestep Index"=w45, "max step ratio"=w43, "error"=w26, "Method Order"=w29) -> (w38:T1)
      }
    }
    frame True {
      w485 = TRUE ("step accepted?")
      n87 = Bundle By Name(cluster=w483, "step accepted?"=w485, "step complete?"=w485) -> (w484:T1)
    }
  }
  "Simulation data out" <- w5
